vi "New HTTP Session.vi"(6 "verify server (true)":bool, 7 "cookie file":path, 8 "error in (no error)":errorcluster, 9 "password":string, 10 "username":string, 11 "http-client in":refnum<class "httpClient.lvclass">) -> (0 "error out":errorcluster, 3 "http-client out":refnum<class "httpClient.lvclass">)   [LabVIEW 2020, in "httpClient.lvlib" / "httpClient.lvclass"]
uses:
  httpClient.lvclass
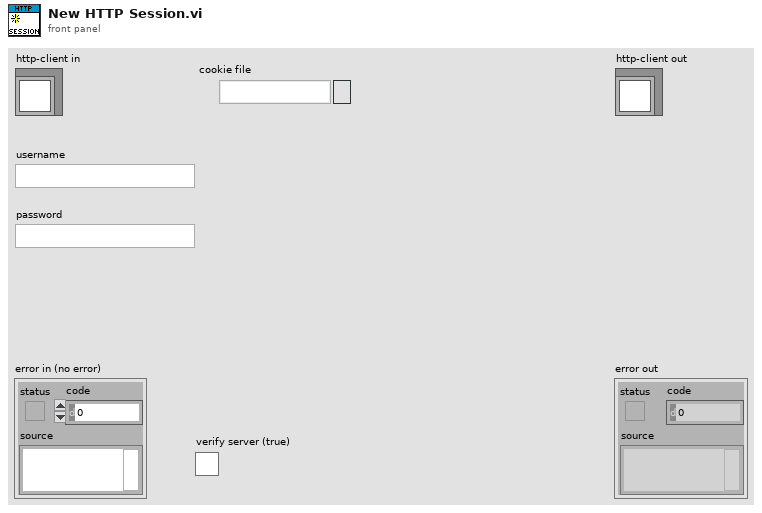
[diagram p1: front panel]
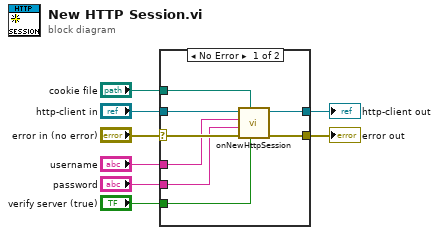
[diagram p0: block diagram]
diagram:
  n1 = case shown="No Error" "error in (no error)" {
    selector: "error in (no error)" -> [w14 w18]
    tunnel: [w13 w18] -> w7
    tunnel: [w16 w17] -> w5
    tunnel: "http-client in" -> [w15 w17]
    tunnel: "username" -> [w12 _]
    tunnel: "password" -> [w11 _]
    tunnel: "verify server (true)" -> [w10 _]
    tunnel: "cookie file" -> [w9 _]
    frame No Error {
      n2 = call-dynamic "onNewHttpSession.vi"("verify server (true)"=w10, "cookie file"=w9, "error in (no error)"=w14, "password"=w11, "username"=w12, "http-client in"=w15) -> ("error out"=w13:errorcluster, "http-client out"=w16:refnum<class "httpClient.lvclass">)  [unwired: 4 in]
    }
    frame Error {
    }
  }
  "error out" <- w7
  "http-client out" <- w5
